vi "GetVI [Poly].vi"   [LabVIEW 2016, in "Drona.lvlib" / "GetVI.lvlib"]
uses:
  GetVI/GetVI.lvlib
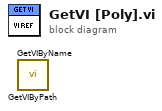
[diagram p0: block diagram]
diagram:
  n1 = call "GetVIByPath.vi"() -> ()  [unwired: 13 in, 3 out]
  n2 = call "GetVIByName.vi"() -> ()  [unwired: 13 in, 3 out]
